vi "Dia 2 - DAQ.vi"() -> ()   [LabVIEW 2014]
uses:
  <vilib>/DAQmx/read.llb/DAQmx Read (Analog DBL 1Chan 1Samp).vi
panel:
  out "XY Graph":cluster{i32[], dbl[]}(graph)
  out "Waveform Chart":dbl(graph)
  in  "Combo Box":string(combo)
  out "String 2":string
  out "K or C":dbl
  out "x/y":dbl
  out "result 2":dbl
  in  "result":dbl
  out "n-1":dbl
  in  "milliseconds to wait":u32
  out "n":dbl format="%0.2f"
  out "data":dbl format="%0.2f"
  in  "stop":bool
  in  "Numeric":i32
  out "Array":dbl[](array[numeric])
  out "data 2":dbl
  in  "DAQmx Task Name":refnum<k21>="RTD"
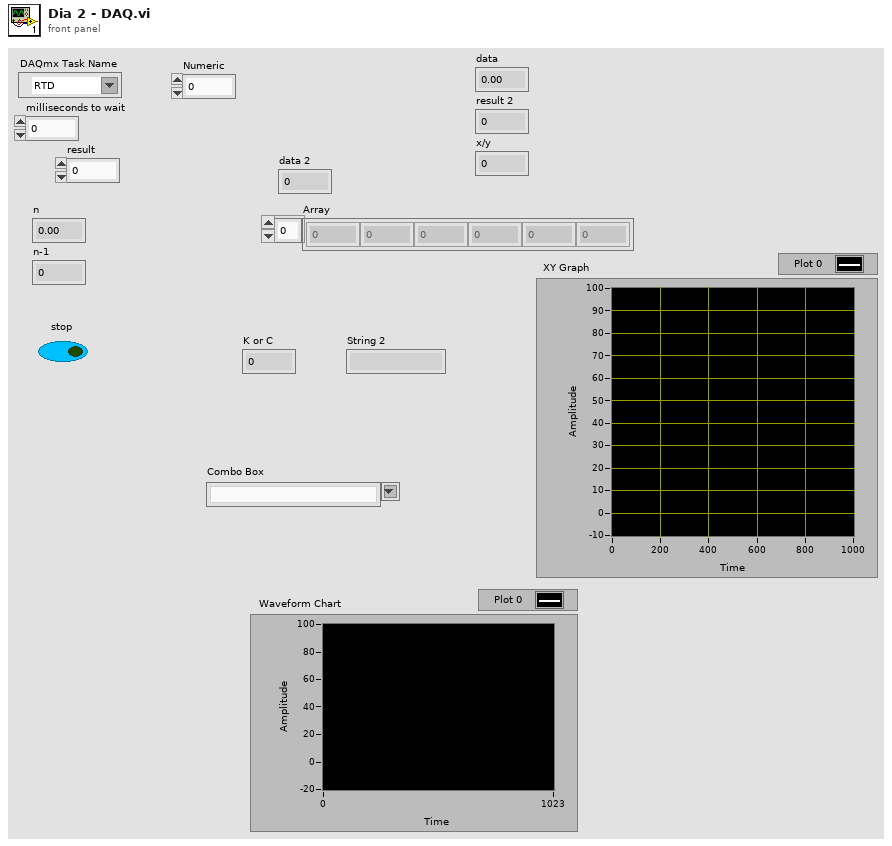
[diagram p1: front panel]
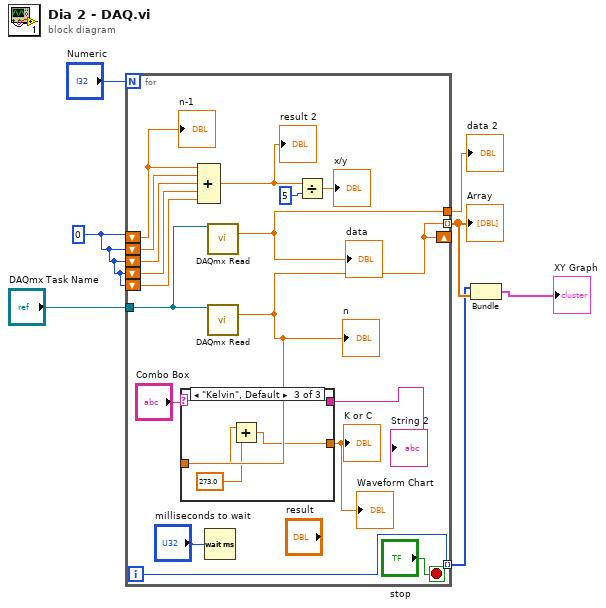
[diagram p0: block diagram]
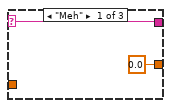
[diagram p2: hidden frame]
diagram:
  w4 = 0
  n1 = for {
    N: "Numeric" -> [_]
    tunnel: "DAQmx Task Name" -> [w23]
    tunnel: [w12] -> w3 mode=indexing
    tunnel: [w22] -> w6
    shift-right: [w12] -> _
    shift-left: w4 -> [w19]
    shift-left: w4 -> [w20]
    shift-left: w4 -> [w18]
    shift-left: w4 -> [w17]
    shift-left: w4 -> [w16]
    tunnel: [w8] -> w2 mode=indexing
    i -> [w8]
    stop <- "stop" stop-if-true
    n2 = Compound Arithmetic op=ADD(w19, w20, w18, w17, w16) -> (w15:dbl)
    "result 2" <- w15
    n3 = Wait (ms)(milliseconds to wait="milliseconds to wait") -> ()  [unwired: 1 out]
    n4 = call-poly <vilib>:"DAQmx Read.vi"("task/channels in"=w23) -> ("data"=w22:dbl)  [unwired: 12 in, 2 out]
    "data" <- w22
    n5 = call-poly <vilib>:"DAQmx Read.vi"("task/channels in"=w23) -> ("data"=w12:dbl)  [unwired: 12 in, 2 out]
    "n" <- w12
    n6 = case shown="\"Kelvin\", Default" "Combo Box" {
      selector: "Combo Box" -> [w25 w27 w29]
      tunnel: w12 -> [_ w28 w32]
      tunnel: [0.0 ("data") w28 w30] -> w9
      tunnel: [w25 w27 w29] -> w11
      frame "Meh" {
      }
      frame "Celsius" {
      }
      frame "Kelvin", Default {
        n7 = Add(x=w32, y=273.0) -> (x+y=w30:dbl)
      }
    }
    "K or C" <- w9
    "String 2" <- w11
    "Waveform Chart" <- w9
    n8 = Divide(x=w15, y=5) -> (x/y=→"x/y":dbl)
    "n-1" <- w19
  }
  "data 2" <- w6
  "Array" <- w3
  n9 = Bundle(w2, w3) -> (→"XY Graph":cluster{i32[], dbl[]})  [unwired: 1 in]
